vi "Config Measure Function.vi"(0 "VISA resource name":refnum<visa-resource-name>, 1 "Autorange (On)":bool=TRUE, 2 "Low Range (1.000)":dbl=1.0, 3 "Range (1.000)":dbl=1.0, 5 "Node In":string, 7 "Channel (Channel A)":T2, 9 "Function (Current)":T1(ring), 11 "error in":errorcluster, 12 "Relative (Off)":bool, 13 "Relative Level (0.000)":dbl) -> (4 "VISA resource name out":refnum<visa-resource-name>, 6 "Node Out":string, 14 "Command String":string, 15 "error out":errorcluster)   [LabVIEW 2009, in "Keithley 2600 Series.lvlib"]
doc: "This VI configures measurement settings that are measure function specific. i.e. Measuring Volts.\n\n<b>Functions and Attributes Used</b>\nsmuX.measure.autorangeY\nsmuX.measure.lowrangeY\nsmuX.measure.rangeY\nsmuX.measure.rel.levelY\nsmuX.measure.rel.enableY"
uses:
  <instrlib>/Keithley 2600 Series/Keithley 2600 Series.lvlib
  <instrlib>/Keithley 2600 Series/Public/Channel.ctl
  <instrlib>/Keithley 2600 Series/Private/GlobalVariables.vi
panel:
  # "(c) 2008 Keithley Instruments, Inc.  ALL RIGHTS RESERVED."
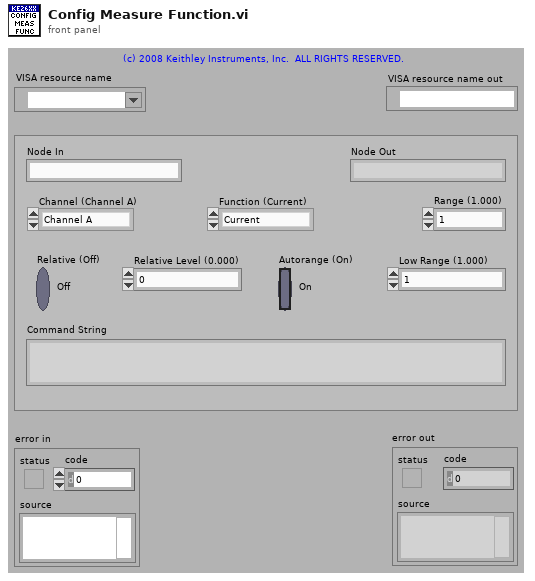
[diagram p1: front panel]
types:
  T1 = enum32{"Current", "Voltage", "Resistance", "Power"}
  T2 = typedef "Keithley 2600 Series.lvlib/Channel.ctl" = enum32{"Channel A", "Channel B"}
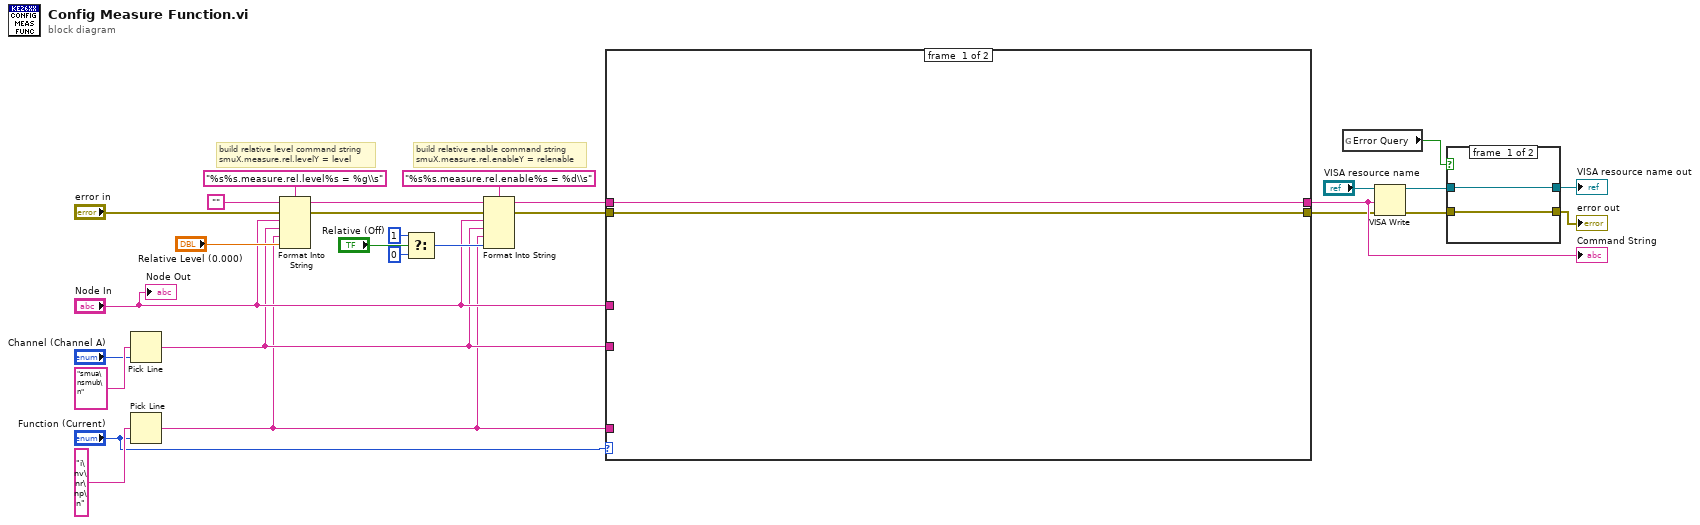
[diagram p0: block diagram]
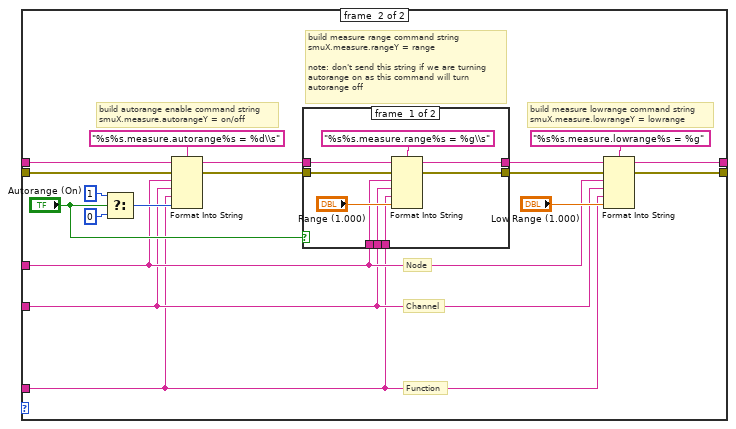
[diagram p2: hidden frame]
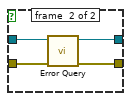
[diagram p4: hidden frame]
diagram:
  # "build relative enable command string\nsmuX.measure.rel.enableY = relenable"
  # "build relative level command string\nsmuX.measure.rel.levelY = level"
  n1 = Pick Line(multi-line string="smua\nsmub\n", line index="Channel (Channel A)") -> (output string=w5:string)  [unwired: 1 out]
  n2 = Pick Line(multi-line string="i\nv\nr\np\n", line index="Function (Current)") -> (output string=w4:string)  [unwired: 1 out]
  n3 = Format Into String(format string="%s%s.measure.rel.level%s = %g\\s", initial string="", error in="error in", "Node In", w5, w4, "Relative Level (0.000)") -> (resulting string=w15:string, error out=w17:errorcluster)
  n4 = Select(t=1, s="Relative (Off)", f=0) -> (s? t:f=w19:i32)
  n5 = Format Into String(format string="%s%s.measure.rel.enable%s = %d\\s", initial string=w15, error in=w17, "Node In", w5, w4, w19) -> (resulting string=w8:string, error out=w7:errorcluster)
  n6 = case shown="\"Current\", \"Voltage\"" "Function (Current)" {
    tunnel: w8 -> [w30 w40]
    tunnel: w7 -> [w29 w39]
    tunnel: "Node In" -> [_ w35]
    tunnel: w5 -> [_ w34]
    tunnel: w4 -> [_ w33]
    tunnel: [w30 w32] -> w3
    tunnel: [w29 w31] -> w2
    frame #0 {
    }
    frame #1 {
      # "build measure lowrange command string\nsmuX.measure.lowrangeY = lowrange"
      # "build measure range command string\nsmuX.measure.rangeY = range\n\nnote: don't send this string if we are turning\nautorange on as this command will turn\nautorange off"
      # "build autorange enable command string\nsmuX.measure.autorangeY = on/off"
      # "Function"
      # "Channel"
      # "Node"
      n7 = Select(t=1, s="Autorange (On)", f=0) -> (s? t:f=w44:i32)
      n8 = Format Into String(format string="%s%s.measure.autorange%s = %d\\s", initial string=w40, error in=w39, w35, w34, w33, w44) -> (resulting string=w42:string, error out=w41:errorcluster)
      n9 = case shown="False" "Autorange (On)" {
        tunnel: w35 -> [w55 _]
        tunnel: w34 -> [w54 _]
        tunnel: w33 -> [w53 _]
        tunnel: w42 -> [w52 w59]
        tunnel: w41 -> [w51 w58]
        tunnel: [w50 w59] -> w37
        tunnel: [w49 w58] -> w36
        frame #0 {
          n10 = Format Into String(format string="%s%s.measure.range%s = %g\\s", initial string=w52, error in=w51, w55, w54, w53, "Range (1.000)") -> (resulting string=w50:string, error out=w49:errorcluster)
        }
        frame #1 {
        }
      }
      n11 = Format Into String(format string="%s%s.measure.lowrange%s = %g", initial string=w37, error in=w36, w35, w34, w33, "Low Range (1.000)") -> (resulting string=w32:string, error out=w31:errorcluster)
    }
  }
  "Command String" <- w3
  n12 = global read "GlobalVariables.vi" "Error Query"() -> (w13:bool)
  n13 = VISA Write(VISA resource name="VISA resource name", write buffer=w3, error in (no error)=w2) -> (VISA resource name out=w12:refnum<visa-resource-name>, error out=w11:errorcluster)  [unwired: 1 out]
  n14 = case shown="True" w13 {
    tunnel: w12 -> [w61 w65]
    tunnel: w11 -> [w60 w64]
    tunnel: [w61 w63] -> w10
    tunnel: [w60 w62] -> w9
    frame #0 {
    }
    frame #1 {
      n15 = call <instrlib>:"Error Query.vi"("error in (no error)"=w64, "VISA resource name"=w65) -> ("error out"=w62:errorcluster, "VISA resource name out"=w63:refnum<visa-resource-name>)  [unwired: 8 out]
    }
  }
  "VISA resource name out" <- w10
  "error out" <- w9
  "Node Out" <- "Node In"
